vi "Prompt for Step--Check for Input.vi"(7 "Control Ref Map":map{string, refnum<vi>}(c390), 8 "error in (no error)":errorcluster, 9 "Macro Hotkey":T1(array[ring]), 10 "Keyboard Ref":refnum<k1>, 11 "Image Assertion in":refnum<class "Image Assertion.lvclass">) -> (0 "error out":errorcluster, 3 "Image Assertion out":refnum<class "Image Assertion.lvclass">)   [LabVIEW 2020, in "MacroAssert.lvlib" / "Image Assertion.lvclass"]
uses:
  Image Assertion.lvclass
  Image Assertion.lvclass/Image Assertion.ctl
  MacroAssert.lvlib
  SubVIs/Win Util/Win Util.lvlib
  Support/Get Control Reference by Label (0D STR).vi
  <vilib>/Utility/miscctls.llb/LVPointTypeDef.ctl
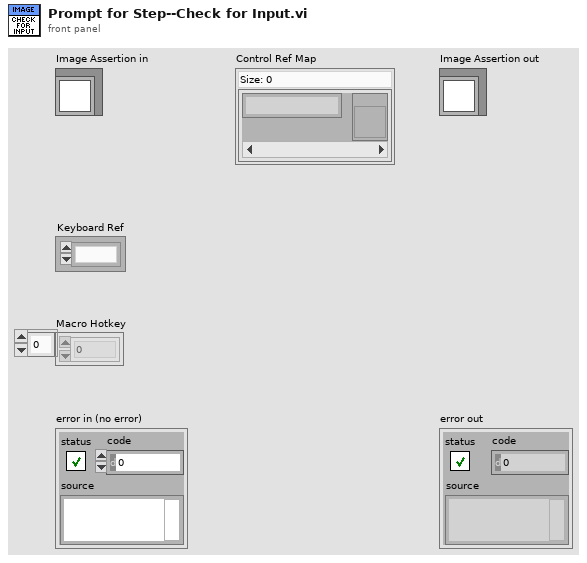
[diagram p1: front panel]
types:
  T1 = enum16{"0", "1", "2", "3", "4", "5", "6", "7", "8", "9", "A", "B", "C", "D", "E", "F", "G", "H", "I", "J", "K", "L", "M", "N", "O", "P", "Q", "R", "S", "T", "U", "V", "W", "X", "Y", "Z", "F1", "F2", "F3", "F4", "F5", "F6", "F7", "F8", "F9", "F10", "F11", "F12", "F13", "F14", "F15", "ADD", "BACK", "BACKSLASH", "CAPITAL", "COMMA", "DECIMAL", "DELETE", "DIVIDE", "DOWN", "END", "EQUALS", "ESCAPE", "GRAVE (`)", "HOME", "INSERT", "LBRACKET", "LCONTROL", "LEFT", "L ALT", "LSHIFT", "LWIN", "MINUS", "MULTIPLY", "NEXT", "NUMLOCK", "NUMPAD_0", "NUMPAD_1", "NUMPAD_2", "NUMPAD_3", "NUMPAD_4", "NUMPAD_5", "NUMPAD_6", "NUMPAD_7", "NUMPAD_8", "NUMPAD_9", "PAUSE", "PERIOD", "PRIOR (PG UP)", "RBRACKET", "RCONTROL", "RETURN", "RIGHT", "R ALT", "RSHIFT", "RWIN", "SCROLL", "SEMICOLON", "SLASH", "SPACE", "SUBTRACT", "TAB", "UP", "ENTER (num pad)", "' (quote)"}[]
  T2 = typedef "LVPointTypeDef.ctl" = cluster{"Horizontal":i16, "Vertical":i16}
  T3 = typedef "MacroAssert.lvlib/Image Assertion.lvclass/Image Units.ctl" = enum16{"Pixels", "Percent"}
  T4 = typedef "MacroAssert.lvlib/Image Assertion.lvclass/Image Assertion Type.ctl" = enum16{"Control Image", "VI Image", "Window Image", "Cursor Icon"}
  T5 = cluster{"left":i16, "top":i16, "right":i16, "bottom":i16}
  T6 = typedef "imagedata.ctl" = cluster{"image type":i32, "image depth":i32, "image":u8[], "mask":u8[], "colors":u32[], "Rectangle":cluster{"left":i16, "top":i16, "right":i16, "bottom":i16}}
  T7 = typedef "MacroAssert.lvlib/Win Util.lvlib/Window Refnum.ctl" = u64
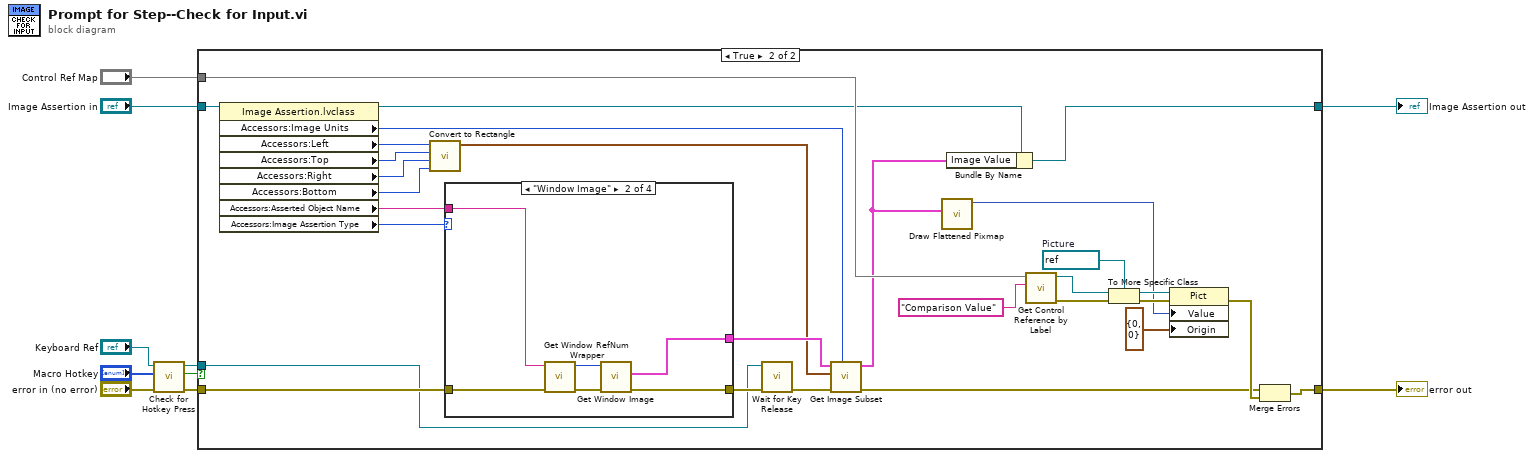
[diagram p0: block diagram]
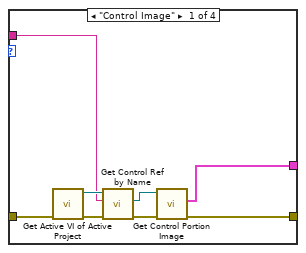
[diagram p3: hidden frame]
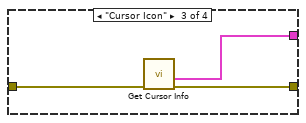
[diagram p4: hidden frame]
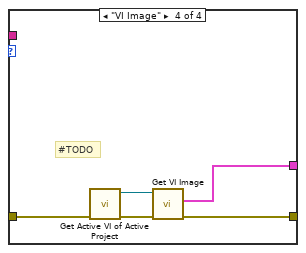
[diagram p5: hidden frame]
diagram:
  n1 = call "Check for Hotkey Press.vi"("error in (no error)"="error in (no error)", "Hotkey"="Macro Hotkey", "Keyboard"="Keyboard Ref") -> ("error out"=w8:errorcluster, "Pressed?"=w3:bool, "Keyboard out"=w6:refnum<k1>)  [unwired: 6 in]
  n2 = case shown="True" w3 {
    tunnel: "Image Assertion in" -> [w11 w20]
    tunnel: [w11 w29] -> w5
    tunnel: w8 -> [w12 w41]
    tunnel: [w12 w40] -> w9
    tunnel: "Control Ref Map" -> [_ w27]
    tunnel: w6 -> [_ w32]
    frame False {
    }
    frame True {
      w30 = refnum<vi> refnum  # Picture
      n3 = property on="Property Node" class="Image Assertion.lvclass"(reference=w20) -> (reference out=w19:refnum<class "Image Assertion.lvclass">, "Accessors:Image Units"=w18:T3, "Accessors:Left"=w21:i16, "Accessors:Top"=w22:i16, "Accessors:Right"=w23:i16, "Accessors:Bottom"=w24:i16, "Accessors:Asserted Object Name"=w16:string, "Accessors:Image Assertion Type"=w15:T4)  [unwired: 1 in, 1 out]
      n4 = call "Convert to Rectangle.vi"("Bottom"=w24, "Right"=w23, "Top"=w22, "Left"=w21) -> ("Rectangle"=w17:T5)  [unwired: 7 in]
      n5 = case shown="\"Window Image\"" w15 {
        tunnel: w41 -> [w47 w55 w58 w63]
        tunnel: [w46 w53 w57 w61] -> w38
        tunnel: w16 -> [w43 w52 _ _]
        tunnel: [w42 w50 w56 w59] -> w25
        frame "Control Image" {
          n6 = call "Get Active VI of Active Project.vi"("error in (no error)"=w47) -> ("error out"=w49:errorcluster, "Active VI Ref"=w45:refnum<vi>)  [unwired: 9 in]
          n7 = call "Get Control Ref by Name.vi"("error in (no error)"=w49, "Name"=w43, "VI Ref"=w45) -> ("error out"=w48:errorcluster, "Ctl Ref"=w44:refnum<vi>)  [unwired: 6 in, 1 out]
          n8 = call "Get Control Portion Image.vi"("error in (no error)"=w48, "Ctl Ref"=w44) -> ("error out"=w46:errorcluster, "Control Image"=w42:T6)  [unwired: 7 in, 1 out]
        }
        frame "Window Image" {
          n9 = call "Get Window RefNum Wrapper.vi"("error in (no error)"=w55, "Window Name"=w52) -> ("error out"=w54:errorcluster, "window refnum"=w51:T7)  [unwired: 8 in]
          n10 = call "Get Window Image.vi"("error in (no error)"=w54, "window refnum in"=w51) -> ("error out"=w53:errorcluster, "image data"=w50:T6)  [unwired: 7 in, 1 out]
        }
        frame "Cursor Icon" {
          n11 = call "Get Cursor Info.vi"("error in (no error)"=w58) -> ("error out"=w57:errorcluster, "Image"=w56:T6)  [unwired: 6 in, 3 out]
        }
        frame "VI Image" {
          # "#TODO"
          n12 = call "Get Active VI of Active Project.vi"("error in (no error)"=w63) -> ("error out"=w62:errorcluster, "Active VI Ref"=w60:refnum<vi>)  [unwired: 9 in]
          n13 = call "Get VI Image.vi"("error in (no error)"=w62, "VI Ref"=w60) -> ("error out"=w61:errorcluster, "VI Image Data"=w59:T6)  [unwired: 7 in, 1 out]
        }
      }
      n14 = call "Wait for Key Release.vi"("error in (no error)"=w38, "Keyboard"=w32) -> ("error out"=w37:errorcluster)  [unwired: 8 in, 1 out]
      n15 = call "Get Image Subset.vi"("Image Units"=w18, "error in (no error)"=w37, "Rectangle"=w17, "Image"=w25) -> ("error out"=w36:errorcluster, "Image Subset"=w14:T6)  [unwired: 6 in]
      n16 = call <vilib>:"Draw Flattened Pixmap.vi"("image data"=w14) -> ("new picture"=w28:picture)  [unwired: 8 in]
      n17 = Bundle By Name(cluster=w19, "Image Value"=w14) -> (w29:refnum<class "Image Assertion.lvclass">)
      n18 = call-poly "Get Control Reference by Label.vi"("Control Name"="Comparison Value", "Control Ref Map"=w27) -> ("error out"=w35:errorcluster, "Control Ref"=w33:refnum<vi>)  [unwired: 7 in, 1 out]
      n19 = To More Specific Class(target class=w30, reference=w33, error in=w35) -> (specific class reference=w31:refnum<vi>, error out=w34:errorcluster)
      n20 = property class="Pict"(reference=w31, error in=w34, "Value"=w28, "Origin"=T2 {"Horizontal"=0, "Vertical"=0}) -> (error out=w39:errorcluster)  [unwired: 1 out]
      n21 = Merge Errors(w36, w39) -> (w40:errorcluster)
    }
  }
  "error out" <- w9
  "Image Assertion out" <- w5
